vi "LP Globals.vi"() -> ()   [LabVIEW 2015]
uses:
  Controls/RT Streamer Queue element.ctl
  Controls/RT Streamer State.ctl
  Controls/LP Status typedef.ctl
  Controls/Motor Loop Mode Typedef.ctl
  Controls/LP Motor Instruction.ctl
  Controls/LP Motor CMD.ctl
  Controls/LP Axis Closed Loop Data.ctl
  Controls/LP System State Typedef.ctl
  Controls/LP Motor Pos And State.ctl
  Controls/Generic Log Massage.ctl
  Controls/Log Thread Name.ctl
  RT Controls/Generic instruction typedef.ctl
  Controls/LP Motors Status.ctl
  RT Controls/RT Streamer Ack element.ctl
  <vilib>/vision/Image Controls.llb/IMAQ Image.ctl
panel:
  out "Circle":T1
  in  "UpperValue":u8
  out "FrameRec":u16
  out "FrameRate":dbl
  out "Algo Time":u32
  out "RT Video Q":refnum<queue>
  in  "Image":T2
  in  "Yaw Gain":i32=3000
  in  "VelocityY":i32=10000
  out "RollLimit-":bool
  out "PitchLimit-":bool
  out "RollLimit+":bool
  out "PitchLimit+":bool
  in  "Limit R+P-":cluster{"R":dbl, "P":dbl}={"R"=35000.0, "P"=-35000.0}
  in  "Limit R-P-":cluster{"R":dbl, "P":dbl}={"R"=-35000.0, "P"=-35000.0}
  in  "Limit R-P+":cluster{"R":dbl, "P":dbl}={"R"=-35000.0, "P"=35000.0}
  in  "Limit R+P+":cluster{"R":dbl, "P":dbl}={"R"=35000.0, "P"=35000.0}
  out "EMGC Stop":bool
  in  "YawOffset":dbl
  in  "RollOffset":dbl
  in  "PitchOffset":dbl
  in  "YawSetpoint":dbl
  in  "RollSetpoint":dbl
  in  "PitchSetpoint":dbl
  out "MotorNotif":refnum<notifier>
  out "StreamOK":bool
  out "ExtendedLogging":bool
  out "Homing@Startup":bool
  in  "RunCurrent":i32=50
  in  "Accelaration":i32=32767
  in  "HoldCurrent":i32=5
  in  "Velocity":i32=10000
  in  "Pitch Gain":i32=3000
  in  "Roll Gain":i32=-3000
  out "YawExist":bool
  in  "HostIP":string="192.168.1.125"
  in  "YawRatio":i32=1
  in  "RollRatio":i32=2144
  in  "PitchRatio":i32=1895
  in  "MotorsStatus":T3
  in  "Sequencer Q":refnum<queue>
  out "Log Q":refnum<queue>
  out "Polling Semaphore":T4
  in  "MotPosition":T5
  out "IMUok":bool
  in  "SysState":T6
  in  "ClosedLoopData":T7
  out "EngageMotors":bool
  in  "Motor Loop Q":refnum<queue>
  in  "MotorLoopMode":T8=enum."Open Loop"
  in  "IMUdata":dbl[](array[numeric])
  out "RT Stream Client Q":refnum<queue>
  in  "LP Status":T9
  out "RT Sreamer Q":refnum<queue>
  # "P 34110\nR 38592"
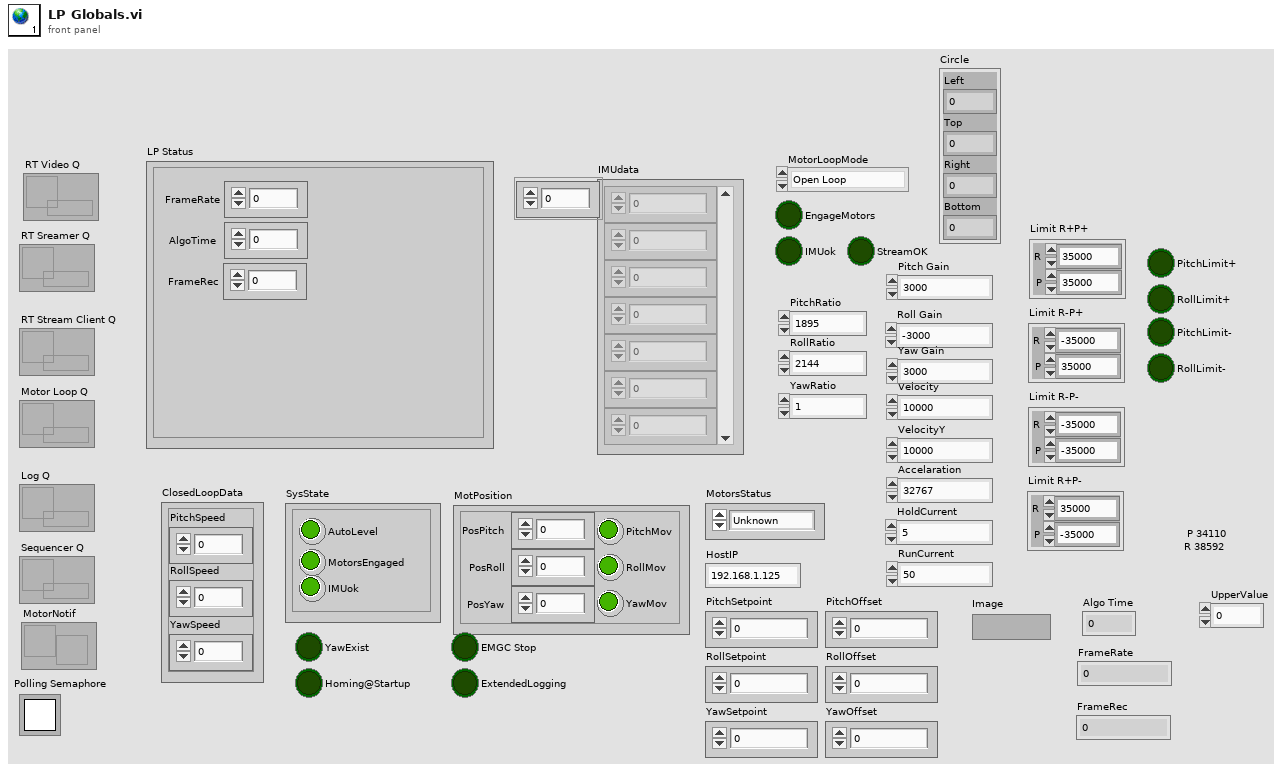
[diagram p1: front panel]
types:
  T1 = cluster{"Left":i32, "Top":i32, "Right":i32, "Bottom":i32}
  T2 = typedef "IMAQ Image.ctl" = refnum<image>
  T3 = typedef "LP Motors Status.ctl" = enum16{"Unknown", "NotHomed", "OK", "Error"}
  T4 = typedef "Semaphore RefNum" = refnum<k1>
  T5 = typedef "LP Motor Pos And State.ctl" = cluster{"PosPitch":dbl, "PosRoll":dbl, "PosYaw":dbl, "PitchMov":bool, "RollMov":bool, "YawMov":bool}
  T6 = typedef "LP System State Typedef.ctl" = cluster{"AutoLevel":bool, "MotorsEngaged":bool, "IMUok":bool}
  T7 = typedef "LP Axis Closed Loop Data.ctl" = cluster{"PitchSpeed":dbl, "RollSpeed":dbl, "YawSpeed":dbl}
  T8 = typedef "Motor Loop Mode Typedef.ctl" = enum16{"NotActive", "Open Loop", "Closed Loop", "ClosedOnce"}
  T9 = typedef "LP Status typedef.ctl" = cluster{"FrameRate":dbl, "AlgoTime":dbl, "FrameRec":u16}
diagram:
